vi "GammaGovernorTarget.vi"() -> ()   [LabVIEW 2014]
uses:
  <vilib>/eio/EIONode/EIONode.xnode
  <vilib>/rvi/eio/common/nirviEmuTemplateMethod_errors.vi
  <vilib>/rvi/DataTransferAndStorage/Container/XNode/niFpgaContainer.xnode
  <vilib>/rvi/interface/RandomDataEmulation/nirviRandomDataFpgaReadWriteTemplate.vi
panel:
  in  "Right reference \nchannel":T1(ring)
  in  "Left reference \nchannel":T1(ring)
  in  "Gamma Module Settings":T2={"35 Hz"=1.0, "55 Hz"=1.0, "75 Hz"=1.0, "95 Hz"=1.0, "Min Cycles"=0, "Max Cycles"=1000, "Phase Select"=enum."Ascending", "Amplitude"=33} {"Amplitude" scale=32.768..32768.0; "95 Hz" scale=0.0..1.0; "75 Hz" scale=0.0..1.0; "55 Hz" scale=0.0..1.0; "35 Hz" scale=0.0..1.0 scale format="%#_2g"}
  in  "Gamma Module Settings":T2={"35 Hz"=1.0, "55 Hz"=1.0, "75 Hz"=1.0, "95 Hz"=1.0, "Min Cycles"=0, "Max Cycles"=1000, "Phase Select"=enum."Ascending", "Amplitude"=33} {"Amplitude" scale=32.768..32768.0; "95 Hz" scale=0.0..1.0; "75 Hz" scale=0.0..1.0; "55 Hz" scale=0.0..1.0; "35 Hz" scale=0.0..1.0 scale format="%#_2g"}
  out "Peak\nAmplitude":i16(slide) scale=32.768..32768.0
  out "Peak\nAmplitude":i16(slide) scale=32.768..32768.0
  in  "Manual left pulse trigger":bool
  in  "Manual right pulse trigger":bool
  in  "Duration":u16
  in  "Timer Stop":bool
  in  "Timer Start":bool
  in  "Toggle Modulation On":bool
  in  "Left Channel Gating Output":refnum<k21>="Connector0/DIO3"
  in  "Left Channel Pulse Output":refnum<k21>="Connector0/DIO1"
  in  "Left channel pulse settings":T3={"Pulse Duration "=2, "Pulse Delay "=0, "Min Pulse Interval"=10}
  in  "Left Gate":bool
  out "Left channel \nstim rate":fxp<+/-,64,32>
  in  "Left channel":i32
  out "Modulation On":bool
  in  "Right Channel Gating Output":refnum<k21>="Connector0/DIO2"
  in  "Right Channel Pulse Output":refnum<k21>="Connector0/DIO0"
  in  "Pulse Gate Digital Input":refnum<k21>="Connector0/DIO4"
  in  "Right channel pulse settings":T3={"Pulse Duration "=2, "Pulse Delay "=0, "Min Pulse Interval"=10}
  in  "Right Gate":bool
  out "Right channel\n stim rate":fxp<+/-,64,32>
  in  "Reset Rate":bool
  out "Host Buffer Overflow":bool
  in  "Right channel":i32
  # "seconds"
  # "Gamma Governor v1.0 \nDrew Headley & Vicky Kanta 2019\nFor research purposes only. \nIf used, please cite:\nKanta, Pare, & Headley, 2019"
  # "Cycle Settings"
  # "Gamma Band Equalizer (% gain)"
  # "Trigger Threshold"
  # "Cycle Settings"
  # "Gamma Band Equalizer (% gain)"
  # "Trigger Threshold"
  # "ms"
  # "ms"
  # "ms"
  # "ms"
  # "ms"
  # "ms"
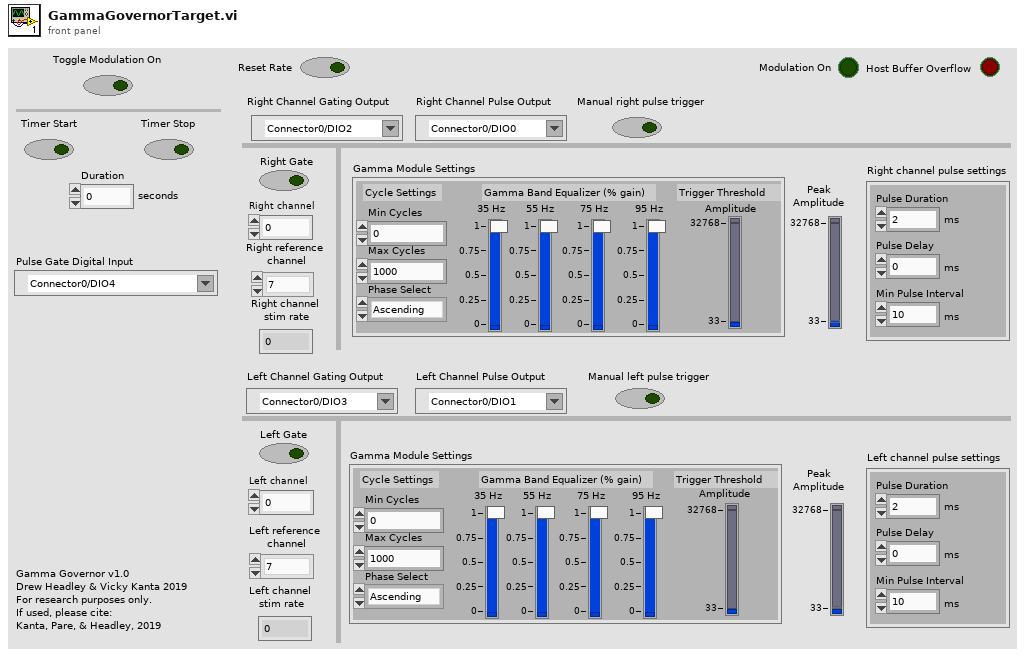
[diagram p1: front panel]
types:
  T1 = enum16{"7", "6", "5", "4", "3", "2", "1", "0", "None"}
  T2 = cluster{"35 Hz":sgl, "55 Hz":sgl, "75 Hz":sgl, "95 Hz":sgl, "Min Cycles":u16, "Max Cycles":u16, "Phase Select":enum16{"Ascending", "Descending", "Peak", "Trough", "Random"}, "Amplitude":i16}
  T3 = cluster{"Pulse Duration ":u32, "Pulse Delay ":u32, "Min Pulse Interval":u16}
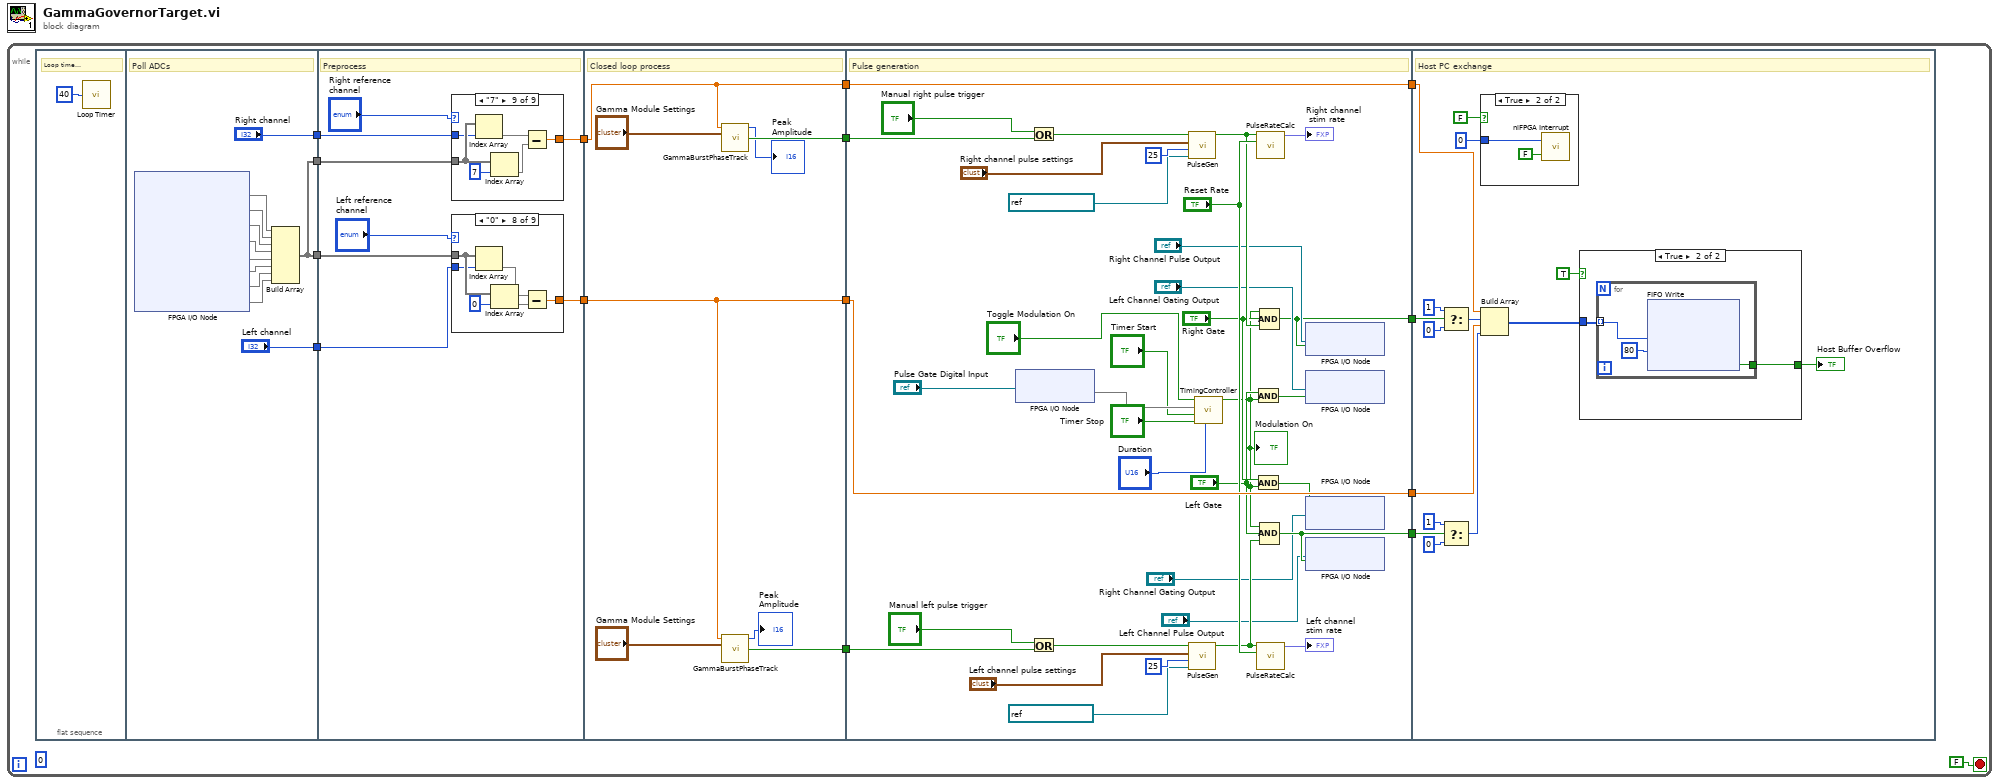
[diagram p0: block diagram]
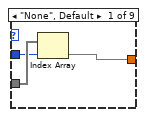
[diagram p2: hidden frame]
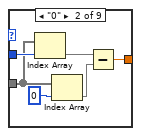
[diagram p3: hidden frame]
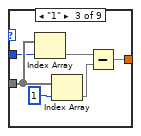
[diagram p4: hidden frame]
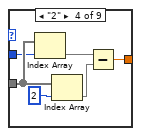
[diagram p5: hidden frame]
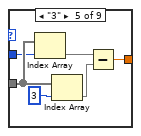
[diagram p6: hidden frame]
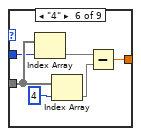
[diagram p7: hidden frame]
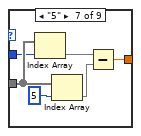
[diagram p8: hidden frame]
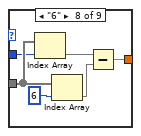
[diagram p9: hidden frame]
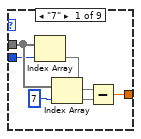
[diagram p10: hidden frame]
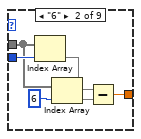
[diagram p11: hidden frame]
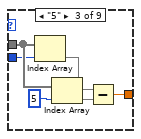
[diagram p12: hidden frame]
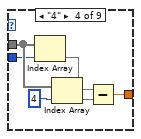
[diagram p13: hidden frame]
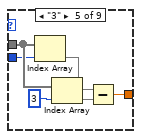
[diagram p14: hidden frame]
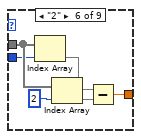
[diagram p15: hidden frame]
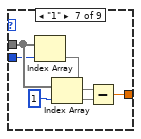
[diagram p16: hidden frame]
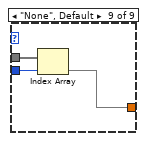
[diagram p17: hidden frame]
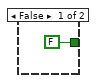
[diagram p19: hidden frame]
diagram:
  n1 = while {
    stop <- FALSE stop-if-true
    (unwired) i16 0
    n2 = flat-sequence {
      tunnel: [w17] -> w14
      tunnel: ["Right channel"] -> w7
      tunnel: ["Left channel"] -> w6
      tunnel: [w17] -> w4
      tunnel: w14 -> [w32]
      tunnel: w7 -> [w29]
      tunnel: w6 -> [w34]
      tunnel: [w33] -> w5
      tunnel: w4 -> [w30]
      tunnel: [w28] -> w3
      tunnel: [w144] -> w13
      tunnel: [w145] -> w11
      tunnel: [w140] -> w9
      tunnel: w5 -> [w140]
      tunnel: w3 -> [w139]
      tunnel: [w139] -> w2
      tunnel: w13 -> [w152]
      tunnel: [w147] -> w12
      tunnel: w11 -> [w149]
      tunnel: [w181] -> w10
      tunnel: w9 -> [w181]
      tunnel: [w171] -> w8
      tunnel: w2 -> [w146]
      tunnel: [w146] -> w1
      tunnel: w12 -> [w191]
      tunnel: w10 -> [w183]
      tunnel: w8 -> [w188]
      tunnel: w1 -> [w182]
      frame #0 {
        # "Loop time\n1 kHz"
        n3 = call "Loop Timer"("Count(uSec)"=u32 40 ("Count(mSec)")) -> ()  [unwired: 1 out]
      }
      frame #1 {
        # "Poll ADCs"
        n4 = xnode "FPGA I/O Node"() -> ("Connector1/AI0"=w27, "Connector1/AI1"=w26, "Connector1/AI2"=w25, "Connector1/AI3"=w24, "Connector1/AI4"=w23, "Connector1/AI5"=w22, "Connector1/AI6"=w21, "Connector1/AI7"=w20)  [unwired: 8 in, 8 out]
        n5 = Build Array(w27, w26, w25, w24, w23, w22, w21, w20) -> (w17:void[])
      }
      frame #2 {
        # "Preprocess"
        n6 = case shown="\"7\"" "Right reference \nchannel" {
          tunnel: w30 -> [w38 w40 w50 w56 w62 w68 w74 w80 w86]
          tunnel: w29 -> [w37 w44 w48 w55 w61 w67 w73 w79 w85]
          tunnel: [w36 w39 w45 w51 w57 w63 w69 w75 w81] -> w28
          frame "None", Default {
            n7 = Index Array(array=w38, index=w37) -> (element=w36)
          }
          frame "0" {
            n8 = Index Array(array=w40, index=w44) -> (element=w42)
            n9 = Index Array(array=w40, index=0) -> (element=w41)
            n10 = Subtract(x=w42, y=w41) -> (x-y=w39:dbl)
          }
          frame "1" {
            n11 = Index Array(array=w50, index=w48) -> (element=w47)
            n12 = Index Array(array=w50, index=1) -> (element=w46)
            n13 = Subtract(x=w47, y=w46) -> (x-y=w45:dbl)
          }
          frame "2" {
            n14 = Index Array(array=w56, index=w55) -> (element=w53)
            n15 = Index Array(array=w56, index=2) -> (element=w52)
            n16 = Subtract(x=w53, y=w52) -> (x-y=w51:dbl)
          }
          frame "3" {
            n17 = Index Array(array=w62, index=w61) -> (element=w59)
            n18 = Index Array(array=w62, index=3) -> (element=w58)
            n19 = Subtract(x=w59, y=w58) -> (x-y=w57:dbl)
          }
          frame "4" {
            n20 = Index Array(array=w68, index=w67) -> (element=w65)
            n21 = Index Array(array=w68, index=4) -> (element=w64)
            n22 = Subtract(x=w65, y=w64) -> (x-y=w63:dbl)
          }
          frame "5" {
            n23 = Index Array(array=w74, index=w73) -> (element=w71)
            n24 = Index Array(array=w74, index=5) -> (element=w70)
            n25 = Subtract(x=w71, y=w70) -> (x-y=w69:dbl)
          }
          frame "6" {
            n26 = Index Array(array=w80, index=w79) -> (element=w77)
            n27 = Index Array(array=w80, index=6) -> (element=w76)
            n28 = Subtract(x=w77, y=w76) -> (x-y=w75:dbl)
          }
          frame "7" {
            n29 = Index Array(array=w86, index=w85) -> (element=w83)
            n30 = Index Array(array=w86, index=7) -> (element=w82)
            n31 = Subtract(x=w83, y=w82) -> (x-y=w81:dbl)
          }
        }
        n32 = case shown="\"0\"" "Left reference \nchannel" {
          tunnel: w32 -> [w92 w96 w104 w110 w116 w122 w128 w134 w137]
          tunnel: w34 -> [w87 w97 w102 w109 w115 w121 w127 w133 w136]
          tunnel: [w88 w93 w99 w105 w111 w117 w123 w129 w135] -> w33
          frame "7" {
            n33 = Index Array(array=w92, index=w87) -> (element=w89)
            n34 = Index Array(array=w92, index=7) -> (element=w90)
            n35 = Subtract(x=w89, y=w90) -> (x-y=w88:dbl)
          }
          frame "6" {
            n36 = Index Array(array=w96, index=w97) -> (element=w95)
            n37 = Index Array(array=w96, index=6) -> (element=w94)
            n38 = Subtract(x=w95, y=w94) -> (x-y=w93:dbl)
          }
          frame "5" {
            n39 = Index Array(array=w104, index=w102) -> (element=w101)
            n40 = Index Array(array=w104, index=5) -> (element=w100)
            n41 = Subtract(x=w101, y=w100) -> (x-y=w99:dbl)
          }
          frame "4" {
            n42 = Index Array(array=w110, index=w109) -> (element=w107)
            n43 = Index Array(array=w110, index=4) -> (element=w106)
            n44 = Subtract(x=w107, y=w106) -> (x-y=w105:dbl)
          }
          frame "3" {
            n45 = Index Array(array=w116, index=w115) -> (element=w113)
            n46 = Index Array(array=w116, index=3) -> (element=w112)
            n47 = Subtract(x=w113, y=w112) -> (x-y=w111:dbl)
          }
          frame "2" {
            n48 = Index Array(array=w122, index=w121) -> (element=w119)
            n49 = Index Array(array=w122, index=2) -> (element=w118)
            n50 = Subtract(x=w119, y=w118) -> (x-y=w117:dbl)
          }
          frame "1" {
            n51 = Index Array(array=w128, index=w127) -> (element=w125)
            n52 = Index Array(array=w128, index=1) -> (element=w124)
            n53 = Subtract(x=w125, y=w124) -> (x-y=w123:dbl)
          }
          frame "0" {
            n54 = Index Array(array=w134, index=w133) -> (element=w131)
            n55 = Index Array(array=w134, index=0) -> (element=w130)
            n56 = Subtract(x=w131, y=w130) -> (x-y=w129:dbl)
          }
          frame "None", Default {
            n57 = Index Array(array=w137, index=w136) -> (element=w135)
          }
        }
      }
      frame #3 {
        # "Closed loop process"
        n58 = call "GammaBurstPhaseTrack.vi"("Input"=w139, "Gamma Module Settings"="Gamma Module Settings") -> ("PeakAmplitude"=→"Peak\nAmplitude":i16, "Phase Trigger"=w144:bool)  [unwired: 10 in, 2 out]
        n59 = call "GammaBurstPhaseTrack.vi"("Input"=w140, "Gamma Module Settings"="Gamma Module Settings") -> ("PeakAmplitude"=→"Peak\nAmplitude":i16, "Phase Trigger"=w145:bool)  [unwired: 10 in, 2 out]
      }
      frame #4 {
        # "Pulse generation"
        n60 = xnode "FPGA I/O Node"("FPGA I/O In"="Pulse Gate Digital Input") -> ("I/O Item"=w170)  [unwired: 1 out]
        n61 = Or(x="Manual right pulse trigger", y=w152) -> (x .or. y?=w153:bool)
        n62 = Or(x="Manual left pulse trigger", y=w149) -> (x .or. y?=w150:bool)
        n63 = call "PulseGen.vi"("Memory"=refnum<k21> "PulseBufferA", "CyclesPerMillisecond"=u16 25 ("TimeFactor"), "Pulse Generator Settings"="Right channel pulse settings", "Trigger"=w153) -> ("PulseOut"=w173:bool)  [unwired: 6 in, 1 out]
        n64 = call "PulseGen.vi"("Memory"=refnum<k21> "PulseBufferB", "CyclesPerMillisecond"=u16 25, "Pulse Generator Settings"="Left channel pulse settings", "Trigger"=w150) -> ("PulseOut"=w172:bool)  [unwired: 6 in, 1 out]
        n65 = call "TimingController.vi"("Duration"="Duration", "Timer Stop"="Timer Stop", "Timer Start"="Timer Start", "InputGate"=w170, "Toggle Modulation On"="Toggle Modulation On") -> ("Running"=w158:bool)  [unwired: 6 in]
        "Modulation On" <- w158
        n66 = And(x="Left Gate", y=w158) -> (x .and. y?=w164:bool)
        n67 = And(x="Right Gate", y=w158) -> (x .and. y?=w166:bool)
        n68 = call "PulseRateCalc.vi"("ResetRate"="Reset Rate", "TriggerIn"=w173) -> ("RateOut"=→"Right channel\n stim rate":fxp<+/-,64,32>)  [unwired: 9 in]
        n69 = call "PulseRateCalc.vi"("ResetRate"="Reset Rate", "TriggerIn"=w172) -> ("RateOut"=→"Left channel \nstim rate":fxp<+/-,64,32>)  [unwired: 9 in]
        n70 = Compound Arithmetic op=AND(w158, "Right Gate", w173) -> (w147:bool)
        n71 = Compound Arithmetic op=AND(w158, "Left Gate", w172) -> (w171:bool)
        n72 = xnode "FPGA I/O Node"("I/O Item"=w147, "FPGA I/O In"="Right Channel Pulse Output") -> ()  [unwired: 1 out]
        n73 = xnode "FPGA I/O Node"("I/O Item"=w164, "FPGA I/O In"="Left Channel Gating Output") -> ()  [unwired: 1 out]
        n74 = xnode "FPGA I/O Node"("I/O Item"=w166, "FPGA I/O In"="Right Channel Gating Output") -> ()  [unwired: 1 out]
        n75 = xnode "FPGA I/O Node"("I/O Item"=w171, "FPGA I/O In"="Left Channel Pulse Output") -> ()  [unwired: 1 out]
      }
      frame #5 {
        # "Host PC exchange"
        n76 = Select(t=i16 1, s=w191, f=i16 0) -> (s? t:f=w185:i16)
        n77 = Select(t=i16 1, s=w188, f=i16 0) -> (s? t:f=w187:i16)
        n78 = case shown="True" FALSE {
          tunnel: u8 0 ("IRQ Number (0)") -> [_ w197]
          frame False {
          }
          frame True {
            n79 = call <vilib>:"niFPGA Interrupt.vi"("Wait Until Cleared (F)"=FALSE, "IRQ Number (0)"=w197) -> ()  [unwired: 1 in]
          }
        }
        n80 = Build Array(w182, w185, w183, w187) -> (w186:i16[])
        n81 = case shown="True" TRUE {
          tunnel: [FALSE ("Timed Out?") w201] -> w194
          tunnel: w186 -> [_ w200]
          frame False {
          }
          frame True {
            n82 = for {
              tunnel: [w204] -> w201
              tunnel: w200 -> [w203] mode=indexing
              n83 = xnode ("FIFO Write")("Element"=w203, "Timeout"=80) -> ("Timed Out?"=w204:bool)  [unwired: 1 in, 1 out]
            }
          }
        }
        "Host Buffer Overflow" <- w194
      }
    }
  }
